vi "close.vi"(8 "error in (no error)":errorcluster caption="错误输入（无错误）", 11 "TCP 输入":refnum<class "TCP.lvclass">) -> (0 "error out":errorcluster caption="错误输出", 3 "TCP 输出":refnum<class "TCP.lvclass">)   [LabVIEW 2016, in "潮位站数据传输.lvlib" / "TCP.lvclass"]
uses:
  TCP.lvclass
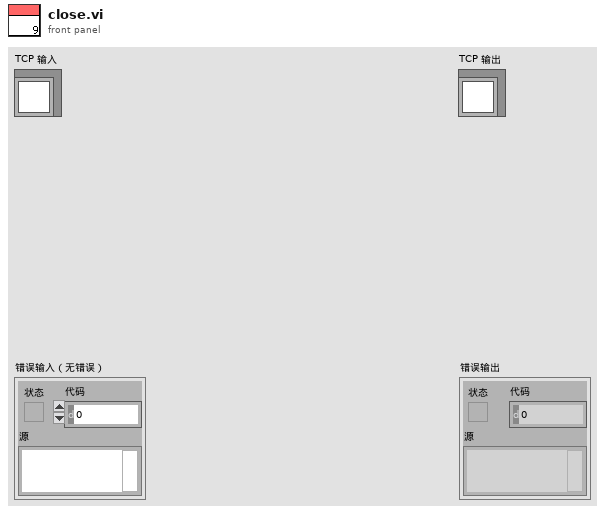
[diagram p1: front panel]
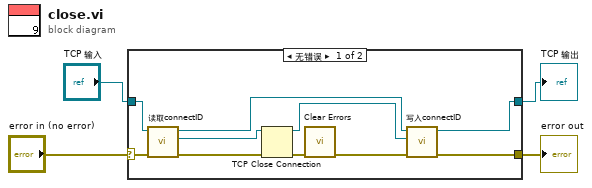
[diagram p0: block diagram]
diagram:
  n1 = case shown="无错误" "error in (no error)" {
    selector: "error in (no error)" -> [w6 w16]
    tunnel: "TCP 输入" -> [w12 w15]
    tunnel: [w10 w15] -> w3
    tunnel: [w8 w16] -> w2
    frame No Error {
      n2 = call-dynamic "读取connectID.vi"("error in (no error)"=w6, "data_inter输入"=w12) -> ("error out"=w5:errorcluster, "connectID"=w13:refnum<k5>, "data_inter输出"=w7:refnum<class "TCP.lvclass">)  [unwired: 7 in]
      n3 = TCP Close Connection(connection ID=w13, error in (no error)=w5) -> (connection ID out=w11:refnum<k5>, error out=w14:errorcluster)  [unwired: 1 in]
      n4 = call <vilib>:"Clear Errors.vi"("error in (no error)"=w14) -> ("error out"=w9:errorcluster)  [unwired: 5 in, 1 out]
      n5 = call-dynamic "写入connectID.vi"("error in (no error)"=w9, "connectID"=w11, "data_inter输入"=w7) -> ("error out"=w8:errorcluster, "data_inter输出"=w10:refnum<class "TCP.lvclass">)  [unwired: 7 in]
    }
    frame Error {
    }
  }
  "error out" <- w2
  "TCP 输出" <- w3
